vi "打开串口.vi"(8 "Error in":errorcluster caption="Error in (no error)") -> (0 "Error out":errorcluster)   [LabVIEW 2016, in "NAQ_DO.lvlib"]
uses:
  NAQ_DO.lvlib
  <vilib>/Plasmionique/MB Master/MB_Master_Serial/MB_Master_Serial.lvclass
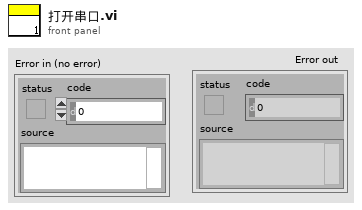
[diagram p1: front panel]
types:
  T1 = cluster{"baud rate (bps)":u32, "stop bits":u16, "parity":u16, "flow control":u16, "timeout":u32, "retries":i32}
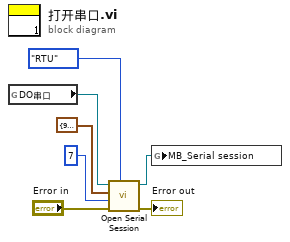
[diagram p0: block diagram]
diagram:
  n1 = global read "过程变量.vi" "DO串口"() -> (w1:refnum<visa-resource-name>)
  n2 = call <vilib>:"Open Serial Session.vi"("Mode (RTU)"=enum16{"RTU", "ASCII"}."RTU", "Error in"="Error in", "Slave ID"=u8 7, "Serial Config"=T1 {"baud rate (bps)"=9600, "stop bits"=10, "parity"=0, "flow control"=0, "timeout"=1000, "retries"=1}, "VISA Resource"=w1) -> ("Error out"=→"Error out":errorcluster, "MB_Serial session"=w2:refnum<class "MB_Master_Serial.lvclass">)  [unwired: 5 in]
  n3 = global write "过程变量.vi" "MB_Serial session"(w2) -> ()
